vi "smooth&reduce.vi"(1 "N-points":i32, 2 "Array in":dbl[](array[numeric]) format="%.2f") -> (0 "Array out":dbl[](array[numeric]) format="%.2f")   [LabVIEW 2013]
uses:
  <vilib>/Analysis/baseanly.llb/Mean (DBL).vi
  <vilib>/Analysis/NI_AALBase.lvlib
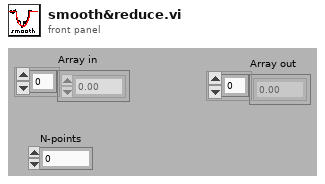
[diagram p1: front panel]
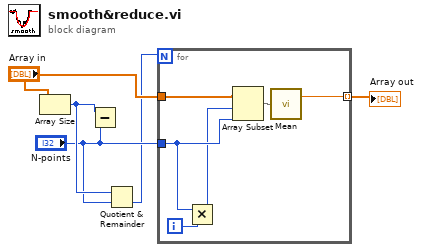
[diagram p0: block diagram]
diagram:
  n1 = Array Size(array="Array in") -> (size(s)=w3:i32)
  n2 = Subtract(x=w3, y="N-points") -> ()  [unwired: 1 out]
  n3 = Quotient & Remainder(x=w3, y="N-points") -> (floor(x/y)=w1:i32)  [unwired: 1 out]
  n4 = for {
    N: w1 -> [_]
    tunnel: "Array in" -> [w11]
    tunnel: "N-points" -> [w9]
    tunnel: [w6] -> w4 mode=indexing
    i -> [w10]
    n5 = Multiply(x=w9, y=w10) -> (x*y=w8:i32)
    n6 = Array Subset(array=w11, index=w8, length=w9) -> (w7:dbl[])
    n7 = call-poly <vilib>:"Mean.vi"("X"=w7) -> ("mean"=w6:dbl)  [unwired: 1 out]
  }
  "Array out" <- w4
